vi "Get State Subcase.vi"(8 "error in":errorcluster, 11 "State in":string) -> (0 "error out":errorcluster, 1 "State subcase":string, 3 "Parent State":string)   [LabVIEW 2013, in "State Machine Lib.lvlib"]
doc: "Removes a parent state from a hierarchial state"
uses:
  State Machine Lib.lvlib
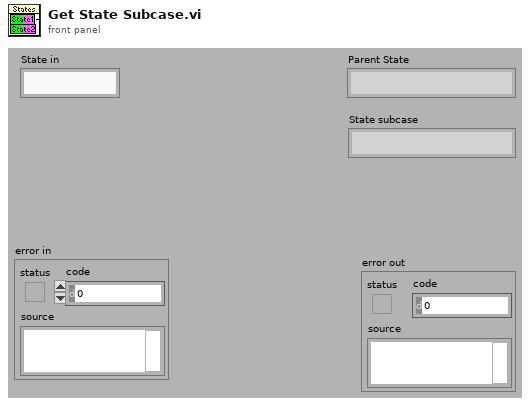
[diagram p1: front panel]
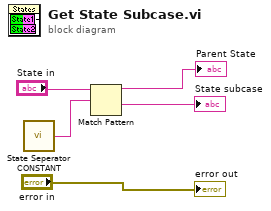
[diagram p0: block diagram]
diagram:
  n1 = call "State Seperator CONSTANT.vi"() -> ("Seperator (:)"=w1:string)
  n2 = Match Pattern(string="State in", regular expression=w1) -> (before substring=→"Parent State":string, after substring=→"State subcase":string)  [unwired: 3 out]
  "error out" <- "error in"
